vi "UI Get time.vi"() -> (1 "Time":dbl, 2 "Time Clusterr":cluster{dbl, dbl, dbl}(knob)={0.0, 55.0, 0.5629564093135127} caption="Timer" scale=0.0..12.0 scale format="%#_1f")   [LabVIEW 2020]
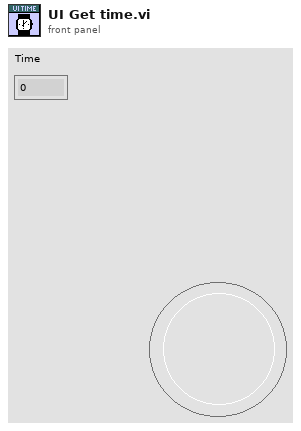
[diagram p1: front panel]
types:
  T1 = typedef "LVDateTimeRec.ctl" = cluster{"fractional second":dbl, "second":i32, "minute":i32, "hour":i32, "day of month":i32, "month":i32, "year":i32, "day of week":i32, "day of year":i32, "DST":i32}
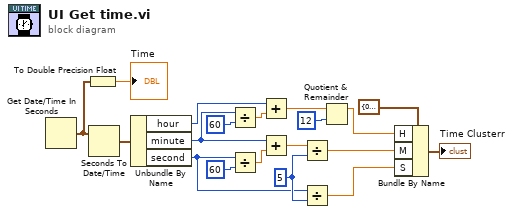
[diagram p0: block diagram]
diagram:
  w13 = 5 ("x")
  n1 = Get Date/Time In Seconds() -> (seconds since 1Jan1904=w2:timestamp)
  n2 = To Double Precision Float(number=w2) -> (double precision float=→"Time":dbl)
  n3 = Seconds To Date/Time(time stamp (now)=w2) -> (date time rec=w19:T1)  [unwired: 1 in]
  n4 = Unbundle By Name(w19) -> ("hour"=w18:i32, "minute"=w10:i32, "second"=w6:i32)
  n5 = Divide(x=w10, y=60) -> (x/y=w7:dbl)
  n6 = Divide(x=w6, y=60) -> (x/y=w3:dbl)
  n7 = Add(x=w18, y=w7) -> (x+y=w8:dbl)
  n8 = Add(x=w10, y=w3) -> (x+y=w4:dbl)
  n9 = Divide(x=w4, y=w13) -> (x/y=w11:dbl)
  n10 = Divide(x=w6, y=w13) -> (x/y=w17:dbl)
  n11 = Quotient & Remainder(x=w8, y=12) -> (x-y*floor(x/y)=w16:dbl)  [unwired: 1 out]
  n12 = Bundle By Name(cluster=cluster{"H":dbl, "M":dbl, "S":dbl} {"H"=0.0, "M"=0.0, "S"=0.0} ("Value"), "H"=w16, "M"=w11, "S"=w17) -> (→"Time Clusterr":cluster{"H":dbl, "M":dbl, "S":dbl})
